vi "Create Project config.vi"(8 "error in (no error)":errorcluster, 10 "Array":refnum<vi>[](array[refnum]), 11 "Refnum in":T1) -> (0 "error out":errorcluster)   [LabVIEW 2018]
doc: "creates ProjectConfig table in existing database."
uses:
  <vilib>/addons/database/Connection.llb/Conn ObjectReference.ctl
  <vilib>/addons/database/Auxilliary.llb/DB Tools Column Info.ctl
  <vilib>/addons/database/Auxilliary.llb/DB Tools DataTypes.ctl
  <vilib>/addons/database/NI_Database_API.lvlib
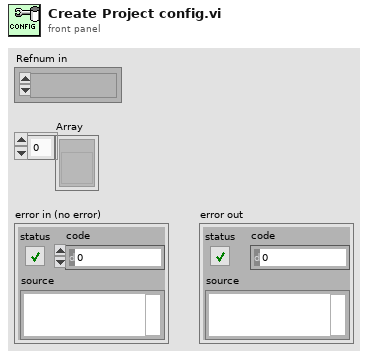
[diagram p1: front panel]
types:
  T1 = typedef "NI_Database_API.lvlib/Conn ObjectReference.ctl" = refnum<k1>
  T2 = typedef "NI_Database_API.lvlib/DB Tools Column Info.ctl" = cluster{"column name":string, "data type":T3, "size":i32, "allow null?":bool}
  T3 = typedef "NI_Database_API.lvlib/DB Tools DataTypes.ctl" = enum16{"String", "Long (I32)", "Single (SGL)", "Double (DBL)", "Date/Time", "Binary"}
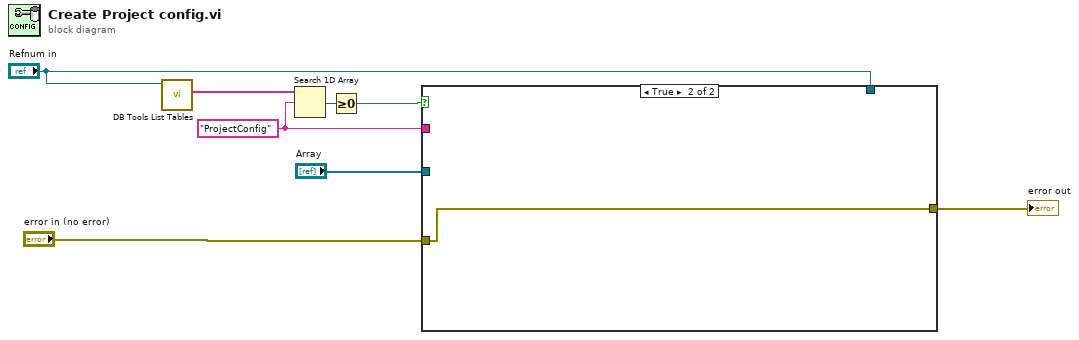
[diagram p0: block diagram]
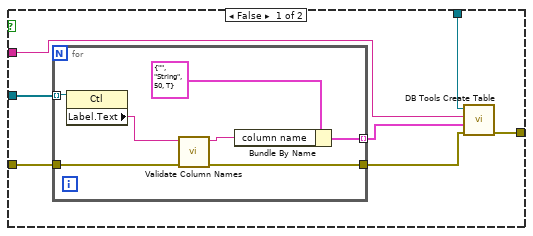
[diagram p2: hidden frame]
diagram:
  w3 = "ProjectConfig" ("table")
  n1 = call <vilib>:"DB Tools List Tables.vi"("connection reference"="Refnum in") -> ("tables"=w4:string[])  [unwired: 4 in, 2 out]
  n2 = Search 1D Array(1D array=w4, element=w3) -> (index of element=w2:i32)  [unwired: 1 in]
  n3 = Greater Or Equal To 0?(x=w2) -> (x >= 0?=w1:bool)
  n4 = case shown="True" w1 {
    tunnel: "Array" -> [w15 _]
    tunnel: "error in (no error)" -> [w13 w23]
    tunnel: [w12 w23] -> w6
    tunnel: "Refnum in" -> [w10 _]
    tunnel: w3 -> [w9 _]
    frame False {
      n5 = for {
        tunnel: w15 -> [w22] mode=indexing
        tunnel: [w20] -> w11 mode=indexing
        tunnel: w13 -> [w18]
        tunnel: [w17] -> w14
        n6 = property class="Ctl"(reference=w22) -> ("Label.Text"=w21:string)  [unwired: 1 in, 2 out]
        n7 = call "Validate Column Names.vi"("error in (no error)"=w18, "Label.Text"=w21) -> ("error out"=w17:errorcluster, "result string"=w19:string)  [unwired: 8 in]
        n8 = Bundle By Name(cluster=T2 {"column name"="", "data type"=enum."String", "size"=50, "allow null?"=TRUE} ("column information"), "column name"=w19) -> (w20:T2)
      }
      n9 = call <vilib>:"DB Tools Create Table.vi"("error in (no error)"=w14, "column information"=w11, "table"=w9, "connection reference"=w10) -> ("error out"=w12:errorcluster)  [unwired: 4 in, 1 out]
    }
    frame True {
    }
  }
  "error out" <- w6
